vi "Verify receiver.vi"(8 "error in (no error)":errorcluster, 10 "Message":string, 11 "RxTxCamera in":refnum<class "RxTxCamera.lvclass">) -> (0 "error out":errorcluster, 2 "verify receiver":bool, 3 "RxTxCamera out":refnum<class "RxTxCamera.lvclass">)   [LabVIEW 2012]
uses:
  RxTxCamera.lvclass
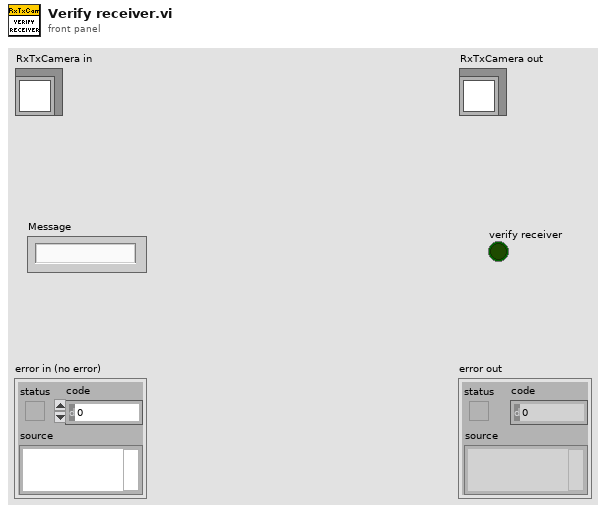
[diagram p1: front panel]
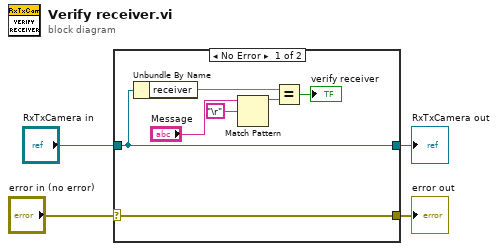
[diagram p0: block diagram]
diagram:
  n1 = case shown="No Error" "error in (no error)" {
    selector: "error in (no error)" -> [w8 w13]
    tunnel: [w8 w13] -> w3
    tunnel: [w6 w12] -> w1
    tunnel: "RxTxCamera in" -> [w6 w12]
    frame No Error {
      n2 = Unbundle By Name(w6) -> ("receiver"=w5)
      n3 = Match Pattern(string="Message", regular expression="\r") -> (before substring=w10:string)  [unwired: 1 in, 3 out]
      n4 = Equal?(x=w5, y=w10) -> (x = y?=→"verify receiver":bool)
    }
    frame Error {
    }
  }
  "error out" <- w3
  "RxTxCamera out" <- w1
